vi "ItemSelection_FireObjectSelectedNotification.vi"(8 "error in (no error)":errorcluster, 10 "Object":T1) -> (0 "error out":errorcluster)   [LabVIEW 2014, in "ItemSelection.lvlib"]
uses:
  ItemSelection.lvlib
  <resource>/Framework/Providers/API/ItemRef.ctl
  ItemSelection_Data.ctl
  ItemSelection_Command.ctl
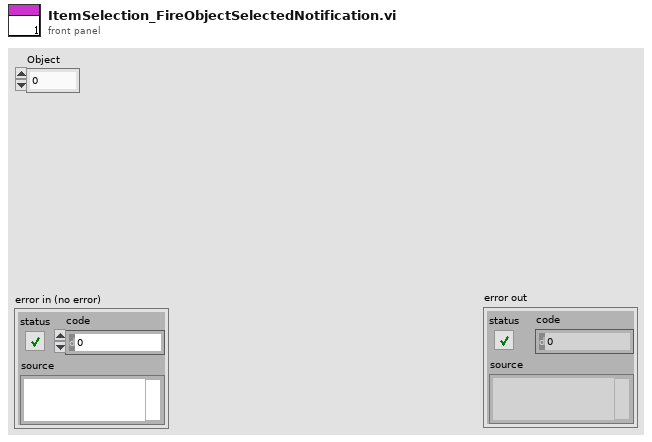
[diagram p1: front panel]
types:
  T1 = typedef "ItemRef.ctl" = u64
  T2 = typedef "ItemSelection.lvlib/ItemSelection_Data.ctl" = cluster{"Command":T3, "Item Ref":T1}
  T3 = typedef "ItemSelection.lvlib/ItemSelection_Command.ctl" = enum16{"ItemSelected", "ItemUnselected"}
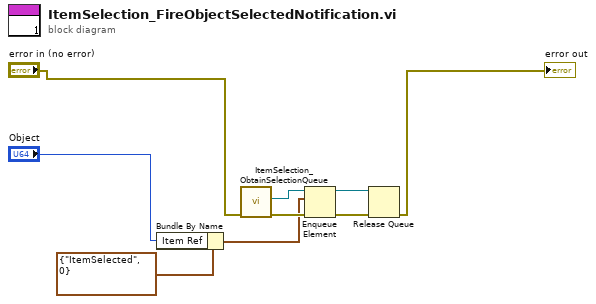
[diagram p0: block diagram]
diagram:
  n1 = Bundle By Name(cluster=T2 {"Command"=enum."ItemSelected", "Item Ref"=0} ("Data"), "Item Ref"="Object") -> (w3:T2)
  n2 = call "ItemSelection_ObtainSelectionQueue.vi"("error in (no error)"="error in (no error)") -> ("error out"=w7:errorcluster, "queue out"=w8:refnum<queue>)  [unwired: 9 in]
  n3 = Enqueue Element(queue=w8, element=w3, error in (no error)=w7) -> (queue out=w5:refnum<queue>, error out=w4:errorcluster)  [unwired: 1 in, 1 out]
  n4 = Release Queue(queue=w5, error in (no error)=w4) -> (error out=→"error out":errorcluster)  [unwired: 1 in, 2 out]
